vi "trace_property_parName_nrChar.vi"(7 "Strings enum":string[](array[string]), 9 "Value enum":u16, 12 "all string":string="all_stringParameters") -> (6 "parameter names":string[](array[string]), 8 "char nr max":i32[](array[numeric]))   [LabVIEW 2010, in "OSA.lvclass"]
uses:
  OSA.lvclass
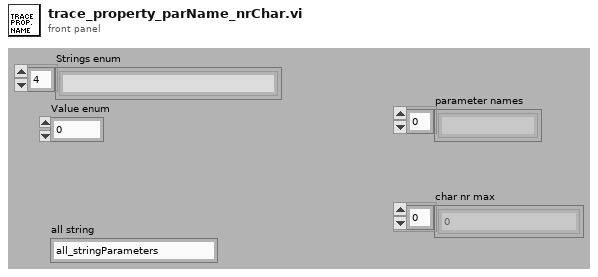
[diagram p1: front panel]
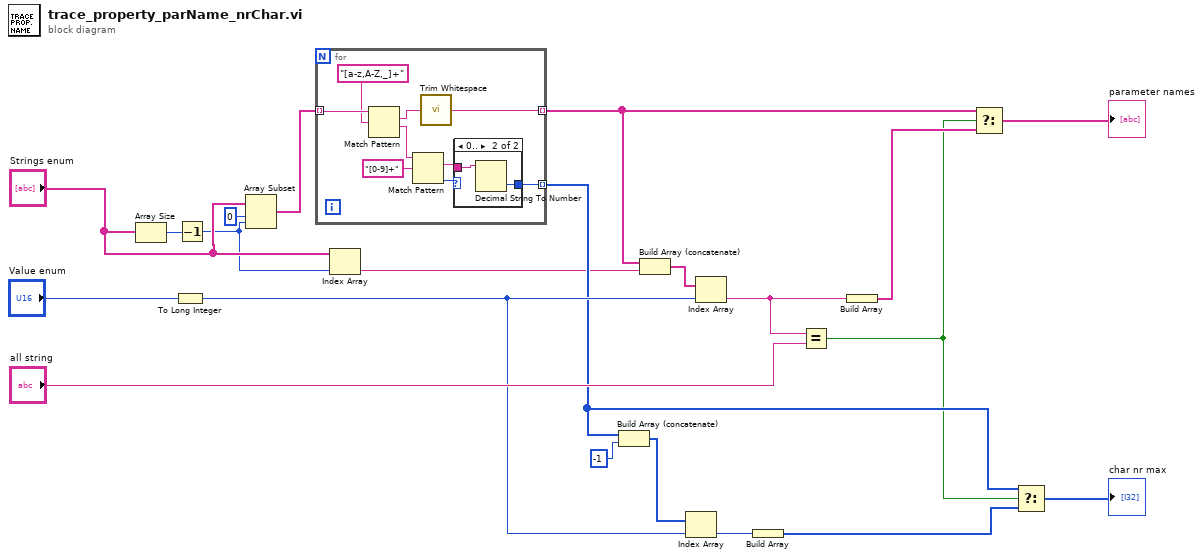
[diagram p0: block diagram]
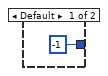
[diagram p2: hidden frame]
diagram:
  n1 = Array Size(array="Strings enum") -> (size(s)=w15:i32)
  n2 = To Long Integer(number="Value enum") -> (32bit integer=w13:i32)
  n3 = Decrement(x=w15) -> (x-1=w4:i32)
  n4 = Array Subset(array="Strings enum", index=0, length=w4) -> (w14:string[])
  n5 = for {
    tunnel: w14 -> [w28] mode=indexing
    tunnel: [w27] -> w1 mode=indexing
    tunnel: [w24] -> w8 mode=indexing
    n6 = Match Pattern(string=w28, regular expression="[a-z,A-Z,_]+") -> (match substring=w26:string, after substring=w30:string)  [unwired: 1 in, 2 out]
    n7 = Match Pattern(string=w30, regular expression="[0-9]+") -> (match substring=w25:string, offset past match=w23:i32)  [unwired: 1 in, 2 out]
    n8 = call <vilib>:"Trim Whitespace.vi"("string"=w26) -> ("trimmed string"=w27:string)  [unwired: 1 in]
    n9 = case shown="0.." w23 {
      tunnel: w25 -> [_ w33]
      tunnel: [-1 w32] -> w24
      frame Default {
      }
      frame 0.. {
        n10 = Decimal String To Number(string=w33) -> (number=w32:i32)  [unwired: 2 in, 1 out]
      }
    }
  }
  n11 = Index Array(array="Strings enum", index=w4) -> (element=w3:string)
  n12 = Build Array (concatenate)(w8, -1 ("number")) -> (w9:i32[])
  n13 = Build Array (concatenate)(w1, w3) -> (w2:string[])
  n14 = Index Array(array=w9, index=w13) -> (element=w11:i32)
  n15 = Index Array(array=w2, index=w13) -> (element=w21:string)
  n16 = Build Array(w11) -> (w10:i32[])
  n17 = Equal?(x=w21, y="all string") -> (x = y?=w7:bool)
  n18 = Build Array(w21) -> (w20:string[])
  n19 = Select(t=w1, s=w7, f=w20) -> (s? t:f=→"parameter names":string[])
  n20 = Select(t=w8, s=w7, f=w10) -> (s? t:f=→"char nr max":i32[])
